vi "1D_Jacobi_eigenvalue_algorithm_v6.vi"() -> ()   [LabVIEW 2020]
uses:
  <vilib>/Analysis/baseanly.llb/Real A x B.vi
  <vilib>/Analysis/baseanly.llb/Mean (DBL).vi
  <vilib>/Analysis/Matrix/Numeric/Conversions/Array To Matrix - RA2.vi
  <vilib>/Analysis/Matrix/Numeric/Conversions/Matrix To Array - RM.vi
  <vilib>/Analysis/7linalg.llb/Real Eigenvalues and Vectors.vi
  <vilib>/Analysis/Matrix/NI_Matrix.lvlib
  <vilib>/Analysis/NI_AALBase.lvlib
  <vilib>/Analysis/NI_AALPro.lvlib
panel:
  out "percent error":dbl
  out "FPGA Jacobi eigenvalue":sgl[](array[numeric])
  in  "Number of Rotations":i32=100
  out "A":dbl[][](array[numeric])
  out "LabVIEW eigvals":dbl[](array[numeric])
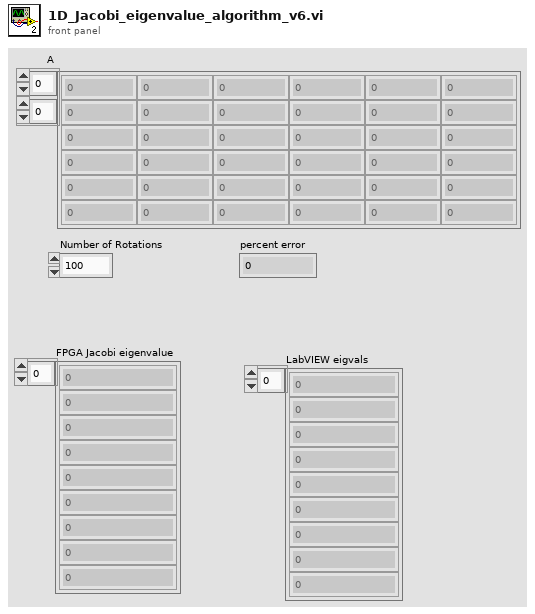
[diagram p1: front panel]
types:
  T1 = typedef "NI_Matrix.lvlib/RealMatrix.ctl" = dbl[][]
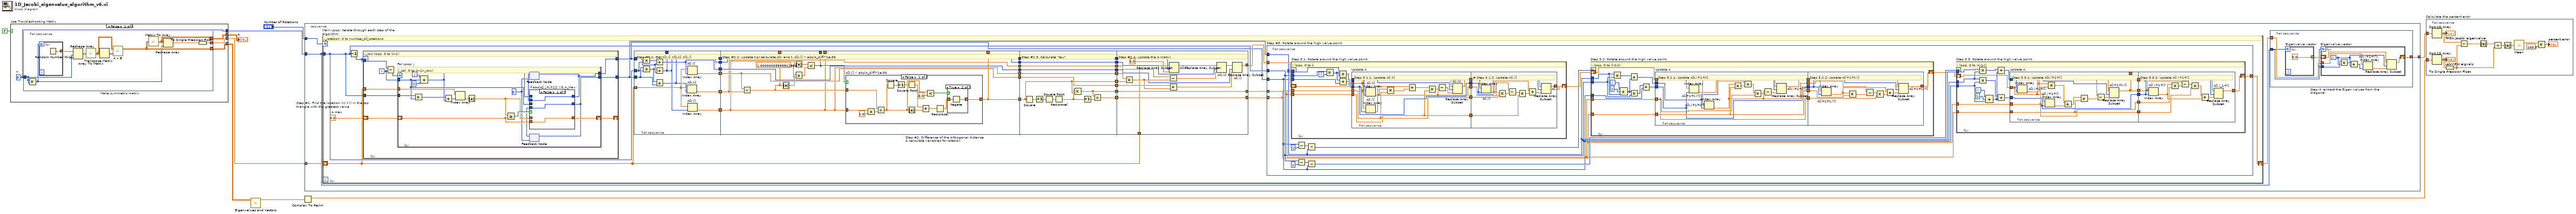
[diagram p0: block diagram]
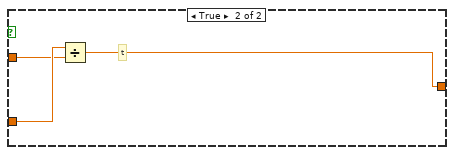
[diagram p3: hidden frame]
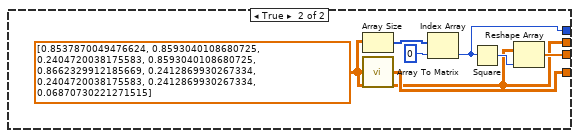
[diagram p5: hidden frame]
diagram:
  n1 = case "Use Troubleshooting Matrix" shown="False" FALSE {
    tunnel: [w12 w31] -> w8
    tunnel: [w13 w30] -> w6
    tunnel: [w11 w28] -> w3
    tunnel: [w10 w25] -> w1
    frame False {
      w10 = 3  # n
      n2 = flat-sequence "Make symmetric matrix" {
        tunnel: [w19] -> w12
        tunnel: [w17] -> w13
        tunnel: [w15] -> w11
        tunnel: w10 -> [w14]
        frame #0 {
          n3 = Multiply(x=w14, y=w14) -> (x*y=w16:i32)
          n4 = for {
            N: w16 -> [_]
            tunnel: [w24] -> w23 mode=indexing
            n5 = Random Number (0-1)() -> (number: 0 to 1=w24:dbl)
          }
          n6 = Reshape Array(w23, w14, w14) -> (w22:dbl[][])
          n7 = call-poly <vilib>:"Array To Matrix.vi"("Real 2D Array"=w22) -> ("Real Matrix"=w21:T1)
          n8 = Transpose Matrix(1:w21) -> (0:w20:T1)
          n9 = call-poly <vilib>:"A x B.vi"("B"=w20, "A"=w21) -> ("A x B"=w19:T1)  [unwired: 1 out]
          n10 = call-poly <vilib>:"Matrix To Array.vi"("Real Matrix"=w19) -> ("Real 2D Array"=w15:dbl[][])
          n11 = Reshape Array(w15, w16) -> (w18:dbl[])
          n12 = To Single Precision Float(number=w18) -> (single precision float=w17:sgl[])
        }
      }
    }
    frame True {
      w28 = sgl[][] [[0.853787, 0.859304, 0.240472], [0.859304, 0.866233, 0.241287], [0.240472, 0.241287, 0.0687073]]
      n13 = Array Size(array=w28) -> (size(s)=w27:i32[])
      n14 = call-poly <vilib>:"Array To Matrix.vi"("Real 2D Array"=w28) -> ("Real Matrix"=w31:T1)
      n15 = Index Array(array=w27, index=0) -> (element=w25:i32)
      n16 = Square(x=w25) -> (x^2=w29:i32)
      n17 = Reshape Array(w28, w29) -> (w30:sgl[])
    }
  }
  "A" <- w3
  n18 = call-poly <vilib>:"Eigenvalues and Vectors.vi"("Input Matrix"=w8) -> ("Eigenvalues"=w9:cdb[])  [unwired: 2 in, 2 out]
  n19 = Complex To Re/Im(x + iy=w9) -> (x=w4:dbl[])  [unwired: 1 out]
  n20 = stacked-sequence {
    tunnel: [w33] -> w5
    tunnel: w1 -> [w32]
    tunnel: "Number of Rotations" -> [w36]
    tunnel: w6 -> [w34]
    frame #0 {
      n21 = for "Main Loop: Iterate through each step of the algorithm" {
        N: w36 -> [_]
        tunnel: w32 -> [w79]
        shift-right: [w50] -> w35
        shift-left: w34 -> [w69]
        w81 = sgl 0.0  # A max
        # "i_rotation: 0 to number_of_rotations"
        n22 = Decrement(x=w79) -> (x-1=w80:i32)
        n23 = for "Step #1: Find the location (in k,l) in the top triangle with the greatest value" {
          N: w80 -> [_]
          tunnel: w80 -> [w299]
          shift-right: [w303] -> _
          shift-left: w81 -> [w301]
          tunnel: [w302] -> w52
          tunnel: [w300] -> w51
          tunnel: w69 -> [w298]
          tunnel: w79 -> [w297]
          i -> [w296]
          # "i_row loop, 0 to (n-1)"
          n24 = Subtract(x=w299, y=w296) -> (x-y=w304:i32)
          n25 = for "For Loop: j" {
            N: w304 -> [_]
            shift-right: [w313] -> w303
            shift-left: w301 -> [w312]
            tunnel: [w305] -> w302
            tunnel: [w309] -> w300
            tunnel: w298 -> [w322]
            tunnel: w296 -> [w311]
            tunnel: w297 -> [w320]
            i -> [w316]
            w306 = 0
            # "j_col, 0 to (n-1-i_row)"
            n26 = Multiply(x=w320, y=w311) -> (x*y=w318:i32)
            n27 = Compound Arithmetic op=ADD(w316, w311, 1 ("value")) -> (w308:i32)
            n28 = Add(x=w318, y=w308) -> (x+y=w317:i32)
            n29 = Index Array(array=w322, index=w317) -> (element=w319:sgl)
            n30 = Absolute Value(x=w319) -> (abs(x)=w314:sgl)
            n31 = Greater Or Equal?(x=w314, y=w312) -> (x >= y?=w315:bool)
            n32 = feedback #1(w306) -> (w307:i32)
            n33 = feedback #2(w306) -> (w310:i32)
            n34 = case "if abs(A[i,j+i+1]) >= A_Max:" shown="False" w315 {
              tunnel: [w325 w328] -> w313
              tunnel: w314 -> [_ w328]
              tunnel: w312 -> [w325 _]
              tunnel: w311 -> [_ w327]
              tunnel: [w324 w327] -> w309
              tunnel: w310 -> [w324 _]
              tunnel: w308 -> [_ w326]
              tunnel: [w323 w326] -> w305
              tunnel: w307 -> [w323 _]
              frame False {
              }
              frame True {
              }
            }
            n35 = feedback-in #1(w305) -> ()
            n36 = feedback-in #2(w309) -> ()
          }
        }
        n37 = flat-sequence "Step #2: Difference of the orthogonal distance & calculate variables for rotation" {
          tunnel: [w89] -> w76
          tunnel: [w88] -> w75
          tunnel: [w87] -> w74
          tunnel: w51 -> [w93]
          tunnel: w79 -> [w92]
          tunnel: w52 -> [w91]
          tunnel: w69 -> [w90]
          tunnel: [w82] -> w65
          tunnel: [w84] -> w64
          tunnel: [w83] -> w61
          tunnel: [w82] -> _
          tunnel: [w97] -> w73
          tunnel: w76 -> [w99]
          tunnel: w75 -> [w98]
          tunnel: w74 -> [w94]
          tunnel: [w102] -> w66
          tunnel: w65 -> [w102]
          tunnel: w64 -> [w101]
          tunnel: [w101] -> w63
          tunnel: w61 -> [w100]
          tunnel: [w100] -> w60
          tunnel: [w94] -> w58
          tunnel: [w99] -> w56
          tunnel: [w98] -> w54
          tunnel: [w97] -> _
          tunnel: [w96] -> _
          tunnel: [w95] -> _
          tunnel: [w94] -> _
          tunnel: w73 -> [w135]
          tunnel: [w135] -> w72
          tunnel: [w134] -> w71
          tunnel: [w133] -> w70
          tunnel: [w132] -> w67
          tunnel: w66 -> [w132]
          tunnel: w63 -> [w131]
          tunnel: [w131] -> w62
          tunnel: w60 -> [w130]
          tunnel: [w130] -> w59
          tunnel: w58 -> [w129]
          tunnel: [w129] -> w57
          tunnel: w56 -> [w128]
          tunnel: [w128] -> w55
          tunnel: w54 -> [w127]
          tunnel: [w127] -> w53
          tunnel: [w156] -> w77
          tunnel: [w157] -> w78
          tunnel: w72 -> [w155]
          tunnel: w71 -> [w157]
          tunnel: w70 -> [w156]
          tunnel: w69 -> [w143]
          tunnel: [w144] -> w68
          tunnel: w67 -> [w150]
          tunnel: w62 -> [w149]
          tunnel: w59 -> [w148]
          tunnel: w57 -> [w147]
          tunnel: w55 -> [w146]
          tunnel: w53 -> [w145]
          frame #0 {
            # "Step #2.1: Get K[I,I], K[k,k], K[k,l]"
            n38 = Multiply(x=w91, y=w92) -> (x*y=w86:i32)
            n39 = Multiply(x=w93, y=w92) -> (x*y=w85:i32)
            n40 = Add(x=w86, y=w91) -> (x+y=w83:i32)
            n41 = Add(x=w85, y=w91) -> (x+y=w82:i32)
            n42 = Add(x=w85, y=w93) -> (x+y=w84:i32)
            n43 = Index Array "A[k,k]"(array=w90, index=w84) -> (element=w88:sgl)
            n44 = Index Array "A[l,l]"(array=w90, index=w83) -> (element=w89:sgl)
            n45 = Index Array "A[k,l]"(array=w90, index=w82) -> (element=w87:sgl)
          }
          frame #1 {
            # "Step #2.2: update t or calculate phi and t, A[k,l] < abs(A_diff)*1e-36"
            n46 = Subtract(x=w99, y=w98) -> (x-y=w96:sgl)
            n47 = Absolute Value(x=w96) -> (abs(x)=w104:sgl)
            n48 = Absolute Value(x=w94) -> (abs(x)=w106:sgl)
            n49 = Multiply(x=w104, y=sgl 1e-36 ("x")) -> (x*y=w105:sgl)
            n50 = Less?(x=w106, y=w105) -> (x < y?=w95:bool)
            n51 = case "A[k,l] < abs(A_diff)*1e-36" shown="False" w95 {
              tunnel: w94 -> [w120 w126]
              tunnel: w96 -> [w117 w125]
              tunnel: [w107 w124] -> w97
              frame False {
                n52 = Multiply(x=w120, y=sgl 2.0) -> (x*y=w118:sgl)
                n53 = Divide(x=w117, y=w118) -> (x/y=w111:sgl)
                n54 = Square(x=w111) -> (x^2=w115:sgl)
                n55 = Increment(x=w115) -> (x+1=w114:sgl)
                n56 = Square Root(x=w114) -> (sqrt(x)=w113:sgl)
                n57 = Absolute Value(x=w111) -> (abs(x)=w116:sgl)
                n58 = Add(x=w113, y=w116) -> (x+y=w112:sgl)
                n59 = Less?(x=w111, y=sgl 0.0) -> (x < y?=w109:bool)
                n60 = Reciprocal(x=w112) -> (1/x=w108:sgl)
                n61 = case shown="True" w109 {
                  tunnel: w108 -> [w121 w123]
                  tunnel: [w121 w122] -> w107
                  frame False {
                  }
                  frame True {
                    n62 = Negate(x=w123) -> (-x=w122:sgl)
                  }
                }
              }
              frame True {
                # "t"
                n63 = Divide(x=w126, y=w125) -> (x/y=w124:sgl)
              }
            }
          }
          frame #2 {
            # "Step #2.3: Calculate \"tau\""
            n64 = Square(x=w135) -> (x^2=w138:sgl)
            n65 = Increment(x=w138) -> (x+1=w137:sgl)
            n66 = Square Root(x=w137) -> (sqrt(x)=w136:sgl)
            n67 = Reciprocal(x=w136) -> (1/x=w140:sgl)
            n68 = Multiply(x=w140, y=w135) -> (x*y=w134:sgl)
            n69 = Increment(x=w140) -> (x+1=w139:sgl)
            n70 = Divide(x=w134, y=w139) -> (x/y=w133:sgl)
          }
          frame #3 {
            # "Step #2.4: update the A matrix"
            n71 = Multiply(x=w147, y=w155) -> (x*y=w154:sgl)
            n72 = Subtract(x=w145, y=w154) -> (x-y=w152:sgl)
            n73 = Add(x=w146, y=w154) -> (x+y=w151:sgl)
            n74 = Replace Array Subset "A[k,l]"(array=w143, new element=sgl 0.0 ("y"), index=w150) -> (w142:sgl[])
            n75 = Replace Array Subset "A[k,k]"(array=w142, new element=w152, index=w149) -> (w141:sgl[])
            n76 = Replace Array Subset "A[l,l]"(array=w141, new element=w151, index=w148) -> (w144:sgl[])
          }
        }
        n77 = flat-sequence "Step #3: Rotate around the high value point" {
          tunnel: w51 -> [w164]
          tunnel: w68 -> [w172]
          tunnel: w79 -> [w165]
          tunnel: w78 -> [w160]
          tunnel: w77 -> [w161]
          tunnel: w52 -> [w163]
          tunnel: [w162] -> w50
          frame #0 {
            n78 = for "Step 3.1: Rotate around the high value point" {
              N: w164 -> [_]
              tunnel: w165 -> [w271]
              tunnel: w164 -> [w270]
              tunnel: w160 -> [w265]
              tunnel: w161 -> [w269]
              tunnel: w163 -> [w266]
              shift-right: [w258] -> w159
              shift-left: w172 -> [w264]
              i -> [w272]
              # "i loop, 0 to k"
              n79 = Multiply(x=w271, y=w272) -> (x*y=w267:i32)
              n80 = Add(x=w267, y=w270) -> (x+y=w263:i32)
              n81 = Add(x=w267, y=w266) -> (x+y=w268:i32)
              n82 = flat-sequence "Update A" {
                tunnel: w269 -> [w276]
                tunnel: w268 -> [w277]
                tunnel: w265 -> [w274]
                tunnel: w264 -> [w280]
                tunnel: w263 -> [w275]
                tunnel: [w278] -> w262
                tunnel: [w277] -> w261
                tunnel: [w276] -> w260
                tunnel: [w274] -> w259
                tunnel: [w273] -> w257
                tunnel: w262 -> [w295]
                tunnel: w261 -> [w287]
                tunnel: w260 -> [w294]
                tunnel: w259 -> [w291]
                tunnel: [w286] -> w258
                tunnel: w257 -> [w285]
                frame #0 {
                  # "Step 3.1.1: Update A[i,k]"
                  n83 = Index Array "A[i,k]"(array=w280, index=w275) -> (element=w273:sgl)
                  n84 = Index Array "A[i,l]"(array=w280, index=w277) -> (element=w283:sgl)
                  n85 = Multiply(x=w273, y=w276) -> (x*y=w284:sgl)
                  n86 = Add(x=w283, y=w284) -> (x+y=w282:sgl)
                  n87 = Multiply(x=w282, y=w274) -> (x*y=w281:sgl)
                  n88 = Subtract(x=w273, y=w281) -> (x-y=w279:sgl)
                  n89 = Replace Array Subset "A[i,k]"(array=w280, new element=w279, index=w275) -> (w278:sgl[])
                }
                frame #1 {
                  # "# Step 3.1.2: Update A[i,l]"
                  n90 = Index Array "A[i,l]"(array=w295, index=w287) -> (element=w289:sgl)
                  n91 = Multiply(x=w289, y=w294) -> (x*y=w293:sgl)
                  n92 = Subtract(x=w285, y=w293) -> (x-y=w292:sgl)
                  n93 = Multiply(x=w292, y=w291) -> (x*y=w290:sgl)
                  n94 = Add(x=w289, y=w290) -> (x+y=w288:sgl)
                  n95 = Replace Array Subset "A[i,l]"(array=w295, new element=w288, index=w287) -> (w286:sgl[])
                }
              }
            }
            n96 = Subtract(x=w163, y=1) -> (x-y=w171:i32)
            n97 = Subtract(x=w165, y=1) -> (x-y=w167:i32)
            n98 = Subtract(x=w171, y=w164) -> (x-y=w169:i32)
            n99 = Subtract(x=w167, y=w163) -> (x-y=w166:i32)
            n100 = for "Step 3.2: Rotate around the high value point" {
              N: w169 -> [_]
              shift-right: [w233] -> w158
              shift-left: w159 -> [w231]
              tunnel: w164 -> [w229]
              tunnel: w165 -> [w225]
              tunnel: w163 -> [w223]
              tunnel: w161 -> [w221]
              tunnel: w160 -> [w219]
              i -> [w228]
              # "i loop, 0 to (l-1-k)"
              n101 = Multiply(x=w229, y=w225) -> (x*y=w227:i32)
              n102 = Compound Arithmetic op=ADD(w228, 1 ("value"), w229) -> (w226:i32)
              n103 = Add(x=w227, y=w226) -> (x+y=w222:i32)
              n104 = Multiply(x=w226, y=w225) -> (x*y=w224:i32)
              n105 = Add(x=w224, y=w223) -> (x+y=w220:i32)
              n106 = flat-sequence "Update A" {
                tunnel: [w245] -> w232
                tunnel: w231 -> [w244]
                tunnel: w222 -> [w236]
                tunnel: w221 -> [w237]
                tunnel: w220 -> [w238]
                tunnel: w219 -> [w235]
                tunnel: [w238] -> w218
                tunnel: [w237] -> w217
                tunnel: [w235] -> w216
                tunnel: [w234] -> w215
                tunnel: [w256] -> w233
                tunnel: w232 -> [w253]
                tunnel: w218 -> [w255]
                tunnel: w217 -> [w254]
                tunnel: w216 -> [w250]
                tunnel: w215 -> [w246]
                frame #0 {
                  # "Step 3.2.1: Update A[k,i+1+k]"
                  n107 = Index Array "A[i+1+k,l?]"(array=w244, index=w238) -> (element=w243:sgl)
                  n108 = Index Array "A[k,i+1+k?]"(array=w244, index=w236) -> (element=w234:sgl)
                  n109 = Multiply(x=w234, y=w237) -> (x*y=w242:sgl)
                  n110 = Add(x=w243, y=w242) -> (x+y=w241:sgl)
                  n111 = Multiply(x=w241, y=w235) -> (x*y=w240:sgl)
                  n112 = Subtract(x=w234, y=w240) -> (x-y=w239:sgl)
                  n113 = Replace Array Subset "A[k,i+1+k?]"(array=w244, new element=w239, index=w236) -> (w245:sgl[])
                }
                frame #1 {
                  # "Step 3.2.2: Update A[i+1+k,l]"
                  n114 = Index Array "A[i+1+k,l?]"(array=w253, index=w255) -> (element=w248:sgl)
                  n115 = Multiply(x=w248, y=w254) -> (x*y=w252:sgl)
                  n116 = Subtract(x=w246, y=w252) -> (x-y=w251:sgl)
                  n117 = Multiply(x=w251, y=w250) -> (x*y=w249:sgl)
                  n118 = Add(x=w248, y=w249) -> (x+y=w247:sgl)
                  n119 = Replace Array Subset "A[i+1+k,l?]"(array=w253, new element=w247, index=w255) -> (w256:sgl[])
                }
              }
            }
            n120 = for "Step 3.3: Rotate around the high value point" {
              N: w166 -> [_]
              tunnel: w165 -> [w187]
              tunnel: w164 -> [w191]
              tunnel: w163 -> [w186]
              shift-right: [w174] -> w162
              shift-left: w158 -> [w182]
              tunnel: w161 -> [w180]
              tunnel: w160 -> [w178]
              i -> [w190]
              # "i loop, 0 to (n-1-l)"
              n121 = Multiply(x=w191, y=w187) -> (x*y=w188:i32)
              n122 = Multiply(x=w187, y=w186) -> (x*y=w185:i32)
              n123 = Compound Arithmetic op=ADD(w190, 1 ("value"), w186) -> (w184:i32)
              n124 = Add(x=w188, y=w184) -> (x+y=w181:i32)
              n125 = Add(x=w185, y=w184) -> (x+y=w179:i32)
              n126 = flat-sequence "Update A" {
                tunnel: [w193] -> w183
                tunnel: w182 -> [w199]
                tunnel: w181 -> [w195]
                tunnel: w180 -> [w196]
                tunnel: w179 -> [w197]
                tunnel: w178 -> [w194]
                tunnel: [w197] -> w177
                tunnel: [w196] -> w176
                tunnel: [w194] -> w175
                tunnel: [w193] -> _
                tunnel: [w192] -> w173
                tunnel: [w214] -> w174
                tunnel: w183 -> [w211]
                tunnel: w177 -> [w213]
                tunnel: w176 -> [w212]
                tunnel: w175 -> [w208]
                tunnel: w173 -> [w204]
                frame #0 {
                  # "Step 3.3.1: Update A[k,i+1+l]"
                  n127 = Index Array "A[k,i+1+l]"(array=w199, index=w195) -> (element=w192:sgl)
                  n128 = Index Array "A[l,i+1+l]"(array=w199, index=w197) -> (element=w202:sgl)
                  n129 = Multiply(x=w192, y=w196) -> (x*y=w203:sgl)
                  n130 = Add(x=w203, y=w202) -> (x+y=w201:sgl)
                  n131 = Multiply(x=w201, y=w194) -> (x*y=w200:sgl)
                  n132 = Subtract(x=w192, y=w200) -> (x-y=w198:sgl)
                  n133 = Replace Array Subset "A[i+1+k,l]"(array=w199, new element=w198, index=w195) -> (w193:sgl[])
                }
                frame #1 {
                  # "Step 3.3.2: Update A[l,i+1+l]"
                  n134 = Index Array "A[l,i+1+l]"(array=w211, index=w213) -> (element=w206:sgl)
                  n135 = Multiply(x=w206, y=w212) -> (x*y=w210:sgl)
                  n136 = Subtract(x=w204, y=w210) -> (x-y=w209:sgl)
                  n137 = Multiply(x=w209, y=w208) -> (x*y=w207:sgl)
                  n138 = Add(x=w207, y=w206) -> (x+y=w205:sgl)
                  n139 = Replace Array Subset "A[l,i_1+l]"(array=w211, new element=w205, index=w213) -> (w214:sgl[])
                }
              }
            }
          }
        }
      }
      n140 = flat-sequence "Step 4: extract the Eigen values from the diagonal" {
        tunnel: w35 -> [w39]
        tunnel: w32 -> [w38]
        tunnel: [w37] -> w33
        frame #0 {
          n141 = for "Eigenvalue vector" {
            N: w38 -> [_]
            tunnel: [sgl 0.0] -> w40 mode=indexing
          }
          n142 = for "Eigenvalue vector" {
            N: w38 -> [_]
            shift-right: [w47] -> w37
            shift-left: w40 -> [w48]
            tunnel: w39 -> [w46]
            tunnel: w38 -> [w45]
            i -> [w43]
            n143 = Multiply(x=w45, y=w43) -> (x*y=w44:i32)
            n144 = Add(x=w44, y=w43) -> (x+y=w42:i32)
            n145 = Index Array "A[k,i+1+l?]"(array=w46, index=w42) -> (element=w41:sgl)
            n146 = Replace Array Subset(array=w48, new element=w41, index=w43) -> (w47:sgl[])
          }
        }
      }
    }
  }
  n147 = flat-sequence "Calculate the percent error" {
    tunnel: w5 -> [w340]
    tunnel: w4 -> [w339]
    frame #0 {
      n148 = Sort 1D Array(array=w340) -> (sorted array=w337:sgl[])
      "FPGA Jacobi eigenvalue" <- w337
      n149 = Sort 1D Array(array=w339) -> (sorted array=w338:dbl[])
      "LabVIEW eigvals" <- w338
      n150 = To Single Precision Float(number=w338) -> (single precision float=w334:sgl[])
      n151 = Subtract(x=w337, y=w334) -> (x-y=w336:sgl[])
      n152 = Absolute Value(x=w336) -> (abs(x)=w335:sgl[])
      n153 = Divide(x=w335, y=w334) -> (x/y=w333:sgl[])
      n154 = Absolute Value(x=w333) -> (abs(x)=w332:sgl[])
      n155 = call-poly <vilib>:"Mean.vi"("X"=w332) -> ("mean"=w331:dbl)  [unwired: 1 out]
      n156 = Multiply(x=w331, y=100.0) -> (x*y=→"percent error":dbl)
    }
  }
